vi "VI Tree.vi"   [LabVIEW 2021, in "Agilent 532XX Series.lvlib"]
doc: "This is the instrument driver for the Agilent 5323XX Series Counter. The VI Tree displays all the user-callable VIs of the instrument driver in an organized table."
uses:
  <instrlib>/Agilent 532XX Series/Agilent 532XX Series.lvlib
  <instrlib>/Agilent 532XX Series/Public/Configure/Measurement/Configure Measurement (Burst).vi
  <instrlib>/Agilent 532XX Series/Public/Configure/Configure Channel (Auto Threshold Voltage).vi
  <instrlib>/Agilent 532XX Series/Public/Data/Read Measurement (Single).vi
  <instrlib>/Agilent 532XX Series/Public/Data/Low Level/Fetch Measurement (Single).vi
panel:
  # "(c) 2010-2015 National Instruments.  ALL RIGHTS RESERVED."
  # "SEE DIAGRAM\nFOR VI TREE."
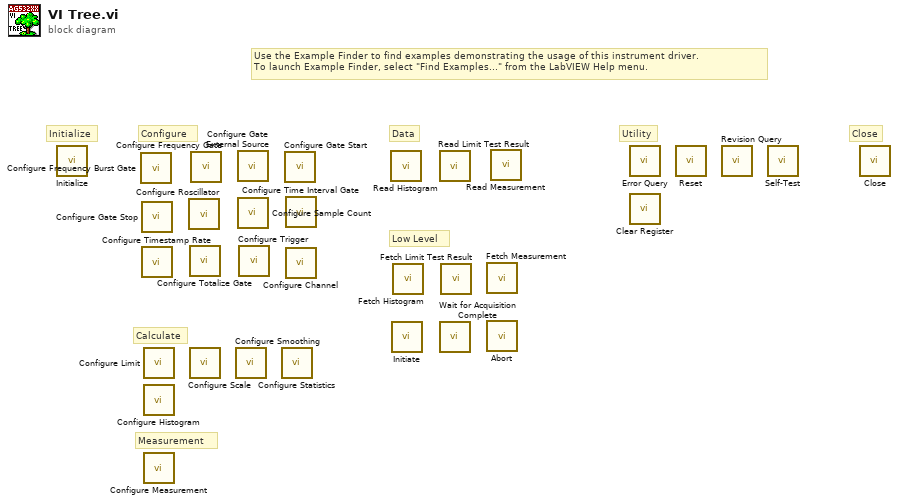
[diagram p0: block diagram]
diagram:
  # "Close"
  # "Utility"
  # "Low Level"
  # "Data"
  # "Measurement"
  # "Calculate"
  # "Configure"
  # "Initialize"
  # "Use the Example Finder to find examples demonstrating the usage of this instrument driver.\nTo launch Example Finder, select \"Find Examples...\" from the LabVIEW Help menu."
  n1 = call <instrlib>:"Initialize.vi"() -> ()  [unwired: 10 in, 2 out]
  n2 = call <instrlib>:"Configure Frequency Burst Gate.vi"() -> ()  [unwired: 10 in, 2 out]
  n3 = call <instrlib>:"Configure Gate Stop.vi"() -> ()  [unwired: 10 in, 2 out]
  n4 = call <instrlib>:"Configure Timestamp Rate.vi"() -> ()  [unwired: 10 in, 2 out]
  n5 = call <instrlib>:"Configure Limit.vi"() -> ()  [unwired: 10 in, 2 out]
  n6 = call <instrlib>:"Configure Histogram.vi"() -> ()  [unwired: 10 in, 2 out]
  n7 = call-poly <instrlib>:"Configure Measurement.vi"() -> ()  [unwired: 10 in, 2 out]
  n8 = call <instrlib>:"Configure Roscillator.vi"() -> ()  [unwired: 10 in, 2 out]
  n9 = call <instrlib>:"Configure Totalize Gate.vi"() -> ()  [unwired: 10 in, 2 out]
  n10 = call <instrlib>:"Configure Scale.vi"() -> ()  [unwired: 14 in, 2 out]
  n11 = call <instrlib>:"Configure Frequency Gate.vi"() -> ()  [unwired: 10 in, 2 out]
  n12 = call <instrlib>:"Configure Smoothing.vi"() -> ()  [unwired: 10 in, 2 out]
  n13 = call <instrlib>:"Configure Gate External Source.vi"() -> ()  [unwired: 10 in, 2 out]
  n14 = call <instrlib>:"Configure Sample Count.vi"() -> ()  [unwired: 10 in, 2 out]
  n15 = call <instrlib>:"Configure Trigger.vi"() -> ()  [unwired: 10 in, 2 out]
  n16 = call <instrlib>:"Configure Statistics.vi"() -> ()  [unwired: 10 in, 2 out]
  n17 = call <instrlib>:"Configure Gate Start.vi"() -> ()  [unwired: 10 in, 2 out]
  n18 = call <instrlib>:"Configure Time Interval Gate.vi"() -> ()  [unwired: 10 in, 2 out]
  n19 = call-poly <instrlib>:"Configure Channel.vi"() -> ()  [unwired: 10 in, 2 out]
  n20 = call <instrlib>:"Read Histogram.vi"() -> ()  [unwired: 6 in, 6 out]
  n21 = call <instrlib>:"Initiate.vi"() -> ()  [unwired: 10 in, 2 out]
  n22 = call <instrlib>:"Fetch Histogram.vi"() -> ()  [unwired: 6 in, 6 out]
  n23 = call <instrlib>:"Read Limit Test Result.vi"() -> ()  [unwired: 8 in, 4 out]
  n24 = call <instrlib>:"Wait for Acquisition Complete.vi"() -> ()  [unwired: 10 in, 2 out]
  n25 = call <instrlib>:"Fetch Limit Test Result.vi"() -> ()  [unwired: 8 in, 4 out]
  n26 = call-poly <instrlib>:"Fetch Measurement.vi"() -> ()  [unwired: 9 in, 3 out]
  n27 = call <instrlib>:"Abort.vi"() -> ()  [unwired: 10 in, 2 out]
  n28 = call-poly <instrlib>:"Read Measurement.vi"() -> ()  [unwired: 9 in, 3 out]
  n29 = call <instrlib>:"Error Query.vi"() -> ()  [unwired: 8 in, 4 out]
  n30 = call <instrlib>:"Clear Register .vi"() -> ()  [unwired: 10 in, 2 out]
  n31 = call <instrlib>:"Reset.vi"() -> ()  [unwired: 10 in, 2 out]
  n32 = call <instrlib>:"Revision Query.vi"() -> ()  [unwired: 8 in, 4 out]
  n33 = call <instrlib>:"Self-Test.vi"() -> ()  [unwired: 8 in, 4 out]
  n34 = call <instrlib>:"Close.vi"() -> ()  [unwired: 11 in, 1 out]
